vi "Main_UI.vi"() -> ()   [LabVIEW 2020]
uses:
  <vilib>/Utility/config.llb/Read Key (I32).vi
  <vilib>/Utility/config.llb/NI_LVConfig.lvlib
panel:
  in  "Start":bool
  in  "Stop":bool
  out "Digital Waveform Graph":digitaldata(graph)
  out "Sampling rate":i32
  out "Channels":i32
  out "Bits":i32
  out "Error out":errorcluster
  in  "Error in":errorcluster
  in  "ADC Type":enum16{"ADC 1", "ADC 2"}(ring)
  # "OBJECTIVE:"
  # "When the VI is run and when the ADC is chosen accordingly the digital data must be displayed in the graph."
  # "INSTRUCTIONS:"
  # "1. Select the ADC required.\n2. Press START button.\n3. The ADC's corresponding Bits, Number of Channels and Sampling rate will be displayed.\n4. The didital data graph will be plotted.\n5. STOP will stop the VI from running."
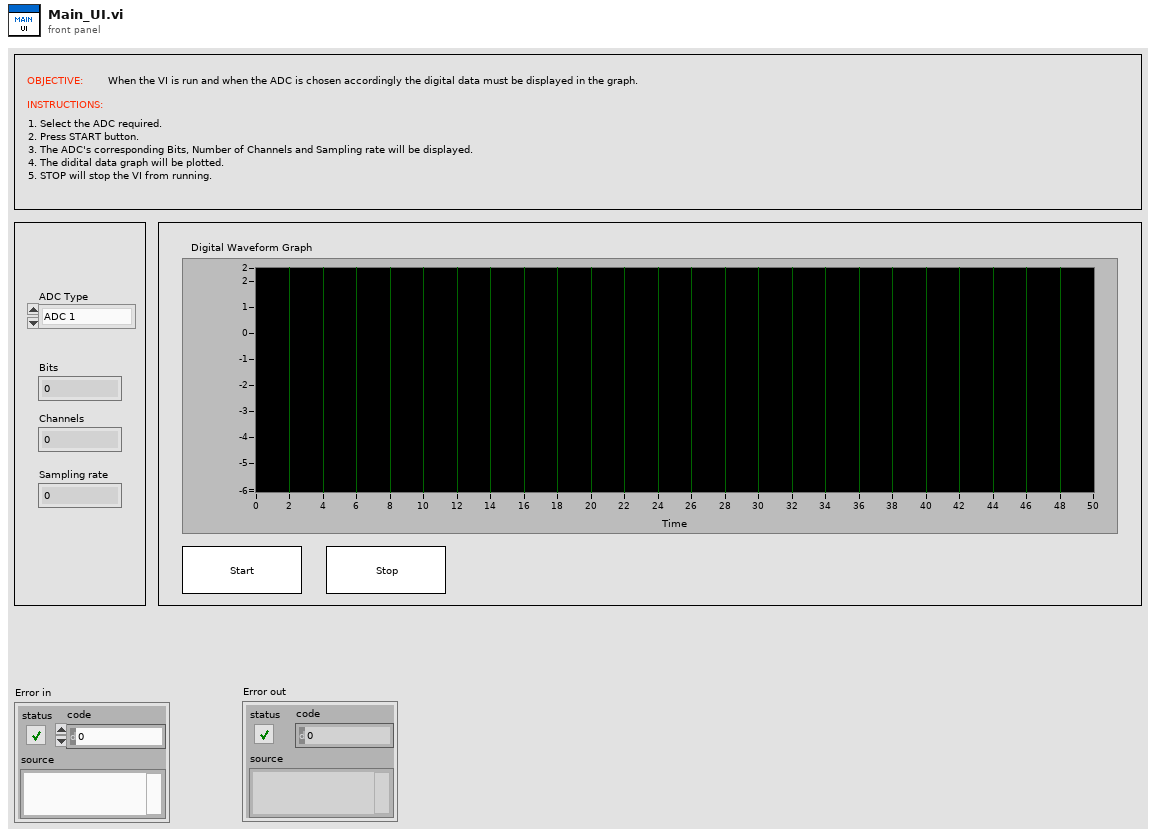
[diagram p1: front panel]
types:
  T1 = typedef "NI_LVConfig.lvlib/Config Data RefNum.ctl" = refnum<k1>
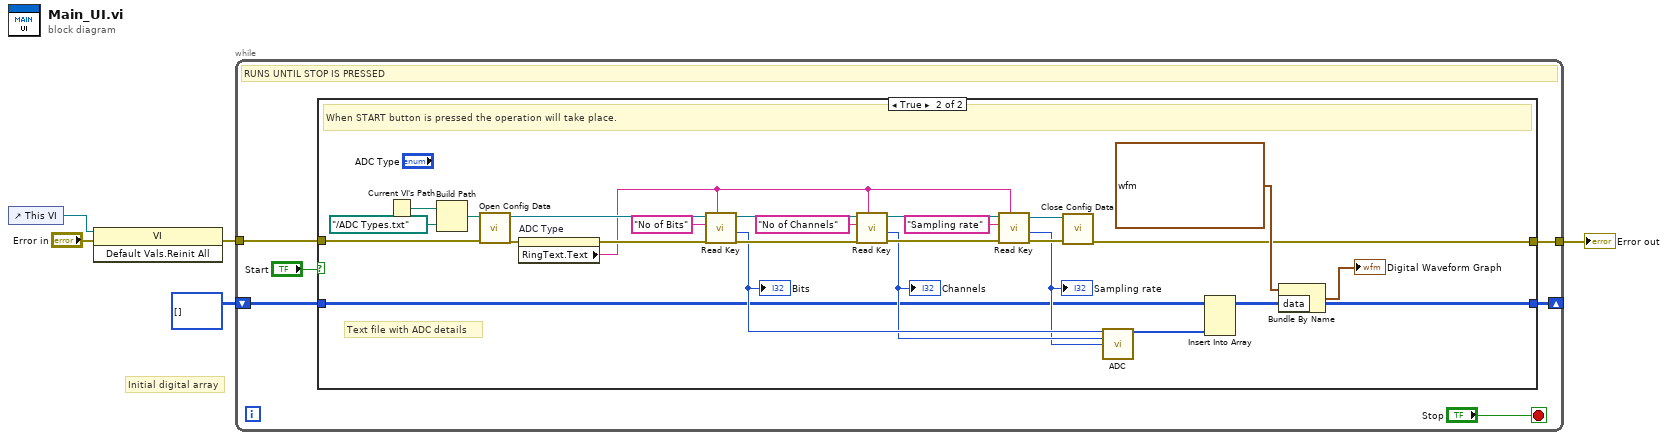
[diagram p0: block diagram]
diagram:
  # "Initial digital array"
  n1 = control-ref of="This VI"() -> (w3:refnum<vi>)
  n2 = invoke class="VI" method="Default Vals.Reinit All"(reference=w3, error in="Error in") -> (error out=w1:errorcluster)  [unwired: 1 in, 2 out]
  n3 = while {
    shift-right: [w10] -> _
    shift-left: u8[][] [] -> [w8]
    tunnel: w1 -> [w9]
    tunnel: [w7] -> w4
    stop <- "Stop" stop-if-true
    # "RUNS UNTIL STOP IS PRESSED"
    n4 = case shown="True" "Start" {
      tunnel: [w12 w17] -> w10
      tunnel: w9 -> [w13 w16]
      tunnel: w8 -> [w12 w15]
      tunnel: [w13 w14] -> w7
      frame False {
        # "Nothing Happens"
      }
      frame True {
        # "Text file with ADC details"
        # "When START button is pressed the operation will take place."
        n5 = Current VI's Path() -> (path=w39:path)
        n6 = Build Path(base path=w39, name or relative path=path "../ADC Types.txt") -> (appended path=w37:path)
        n7 = call <vilib>:"Open Config Data.vi"("error in (no error)"=w16, "configuration file path"=w37) -> ("error out"=w34:errorcluster, "refnum"=w36:T1)  [unwired: 7 in, 1 out]
        n8 = property on="ADC Type" class="Enum (strict)"(error in=w34) -> (error out=w33:errorcluster, "RingText.Text"=w28:string)  [unwired: 1 in, 1 out]
        n9 = call-poly <vilib>:"Read Key.vi"("section"=w28, "error in (no error)"=w33, "key"="No of Bits", "refnum"=w36) -> ("error out"=w24:errorcluster, "value"=w23:i32, "refnum out"=w32:T1)  [unwired: 4 in, 1 out]
        "Bits" <- w23
        n10 = call-poly <vilib>:"Read Key.vi"("section"=w28, "error in (no error)"=w24, "key"="No of Channels", "refnum"=w32) -> ("error out"=w30:errorcluster, "value"=w22:i32, "refnum out"=w29:T1)  [unwired: 4 in, 1 out]
        "Channels" <- w22
        n11 = call-poly <vilib>:"Read Key.vi"("section"=w28, "error in (no error)"=w30, "key"="Sampling rate", "refnum"=w29) -> ("error out"=w26:errorcluster, "value"=w21:i32, "refnum out"=w25:T1)  [unwired: 4 in, 1 out]
        "Sampling rate" <- w21
        n12 = call <vilib>:"Close Config Data.vi"("error in (no error)"=w26, "refnum"=w25) -> ("error out"=w14:errorcluster)  [unwired: 8 in, 1 out]
        n13 = call "ADC.vi"("Bits"=w23, "Channels"=w22, "Sampling rate"=w21) -> ("Digital 1D"=w20:u8[])  [unwired: 12 in]
        n14 = Insert Into Array(array=w15, new element=w20) -> (w17:u8[][])  [unwired: 2 in]
        n15 = Bundle By Name(cluster=digitaldata {"transitions"=[], "data"=[]} ("waveform"), "data"=w17) -> (→"Digital Waveform Graph":digitaldata)
      }
    }
  }
  "Error out" <- w4
